vi "Make number even.vi"(5 "Direction (+Inf)":enum16{"Toward +Inf", "Toward -Inf"}(ring), 6 "Lower limit (0)":i32, 7 "Upper limit (I32 max)":i32=2147483647, 11 "Number in":i32) -> (3 "Even number":i32)   [LabVIEW 2013]
uses:
  <vilib>/GPower/Comparison/Library/IsOdd/IsOddI32.vi
  <vilib>/GPower/Comparison/GPComparison.lvlib
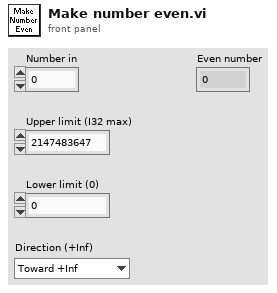
[diagram p1: front panel]
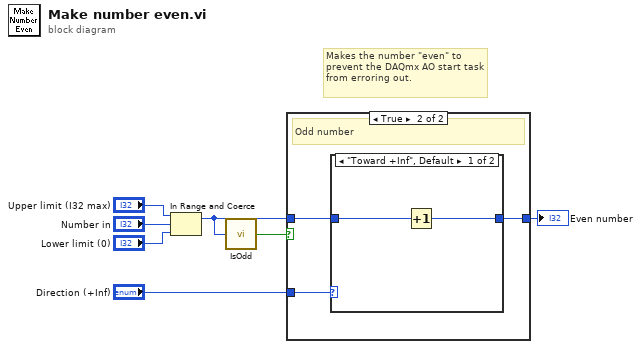
[diagram p0: block diagram]
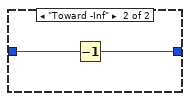
[diagram p3: hidden frame]
diagram:
  # "Makes the number \"even\" to prevent the DAQmx AO start task from erroring out."
  n1 = In Range and Coerce(upper limit="Upper limit (I32 max)", x="Number in", lower limit="Lower limit (0)") -> (coerced(x)=w1:i32)  [unwired: 1 out]
  n2 = call-poly <vilib>:"IsOdd.vi"("x"=w1) -> ("Odd?"=w2:bool)  [unwired: 4 in]
  n3 = case shown="True" w2 {
    tunnel: [w8 w11] -> w4
    tunnel: "Direction (+Inf)" -> [_ w10]
    tunnel: w1 -> [w8 w9]
    frame False {
      # "Even number"
    }
    frame True {
      # "Odd number"
      n4 = case shown="\"Toward +Inf\", Default" w10 {
        tunnel: [w12 w14] -> w11
        tunnel: w9 -> [w13 w15]
        frame "Toward +Inf", Default {
          n5 = Increment(x=w13) -> (x+1=w12:i32)
        }
        frame "Toward -Inf" {
          n6 = Decrement(x=w15) -> (x-1=w14:i32)
        }
      }
    }
  }
  "Even number" <- w4
